vi "ttm_startLogging.vi"(11 "expId":string) -> (1 "loggingOnOut":bool, 2 "startLoggingOut":bool, 3 "expIdOut":string)   [LabVIEW 2009]
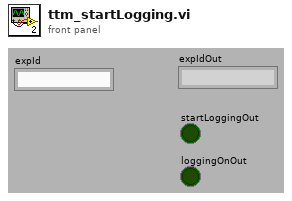
[diagram p1: front panel]
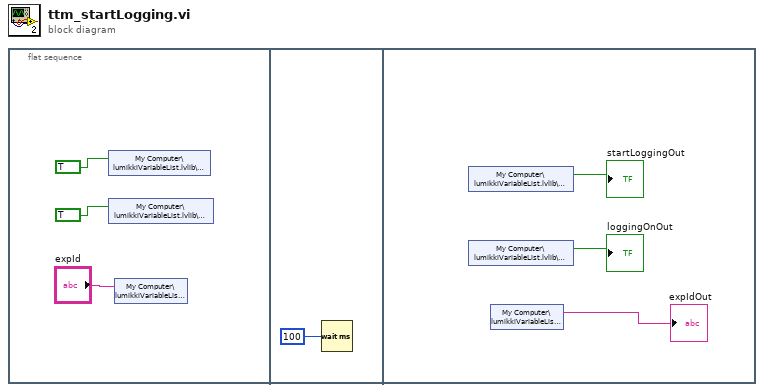
[diagram p0: block diagram]
diagram:
  n1 = flat-sequence {
    frame #0 {
      n2 = shared-variable "My Computer\\lumikkiVariableList.lvlib\\loggingIsOn"(TRUE ("Busy")) -> ()  [unwired: 1 in, 1 out]
      n3 = shared-variable "My Computer\\lumikkiVariableList.lvlib\\startLogging"(TRUE ("Busy")) -> ()  [unwired: 1 in, 1 out]
      n4 = shared-variable "My Computer\\lumikkiVariableList.lvlib\\expId"("expId") -> ()  [unwired: 1 in, 1 out]
    }
    frame #1 {
      n5 = Wait (ms)(milliseconds to wait=u32 100) -> ()  [unwired: 1 out]
    }
    frame #2 {
      n6 = shared-variable "My Computer\\lumikkiVariableList.lvlib\\startLogging"() -> (→"startLoggingOut":bool)  [unwired: 1 in, 1 out]
      n7 = shared-variable "My Computer\\lumikkiVariableList.lvlib\\startLogging"() -> (→"loggingOnOut":bool)  [unwired: 1 in, 1 out]
      n8 = shared-variable "My Computer\\lumikkiVariableList.lvlib\\expId"() -> (→"expIdOut":string)  [unwired: 1 in, 1 out]
    }
  }
